vi "Query Current.vi"(8 "error in (no error)":errorcluster, 11 "VISA resource name":refnum<visa-resource-name>) -> (0 "error out":errorcluster, 1 "Ch2 Motor current (I)":sgl, 2 "Ch1  Motor current (I)":sgl, 3 "VISA resource name out":refnum<visa-resource-name>, 4 "Ch2 Battery current (I)":sgl, 5 "Motor Currents":T1, 6 "Ch1 Battery current (I)":sgl)   [LabVIEW 2011, in "Roboteq.lvlib"]
uses:
  Roboteq.lvlib
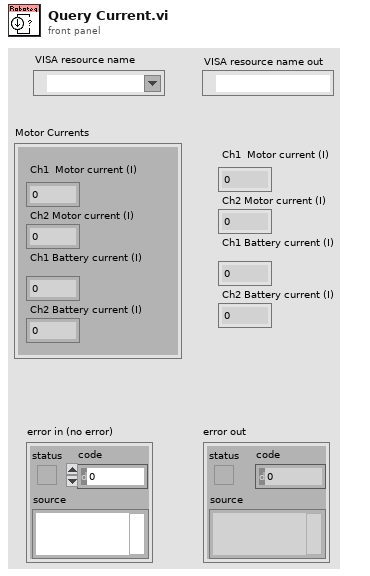
[diagram p1: front panel]
types:
  T1 = cluster{" Ch1  Motor current (I)":sgl, " Ch2 Motor current (I)":sgl, " Ch1 Battery current (I)":sgl, " Ch2 Battery current (I)":sgl}
  T2 = cluster{" Ch1  Motor current (I)":sgl, " Ch2 Motor current (I)":sgl, " Ch1 Battery current (I)":sgl, " Ch2 Battery current (I) 2":sgl}
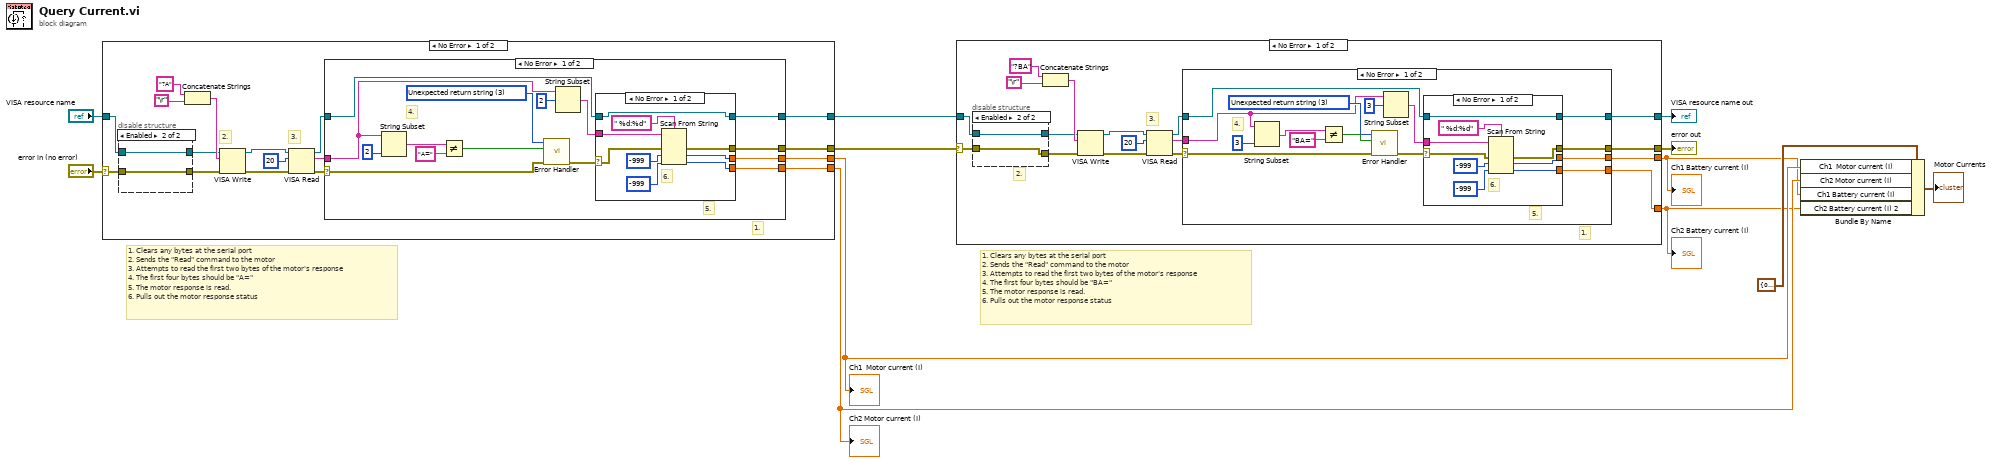
[diagram p0: block diagram]
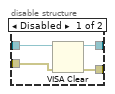
[diagram p2: hidden frame]
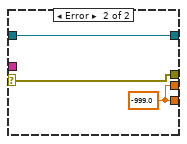
[diagram p3: hidden frame]
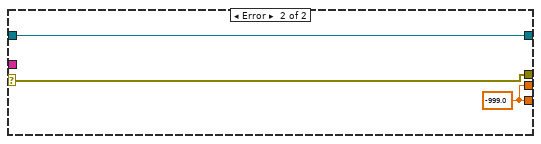
[diagram p4: hidden frame]
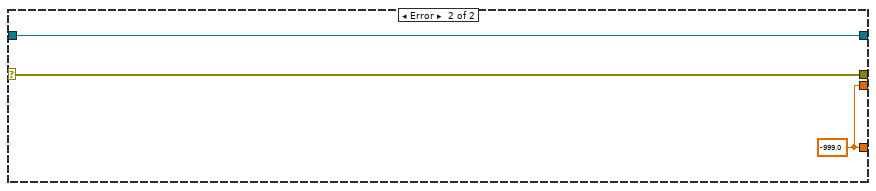
[diagram p5: hidden frame]
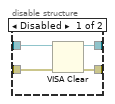
[diagram p6: hidden frame]
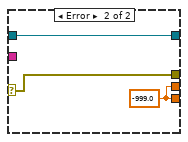
[diagram p7: hidden frame]
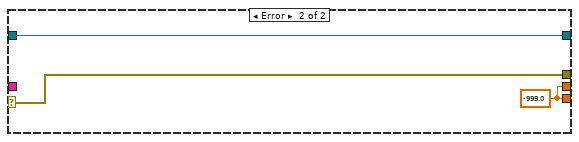
[diagram p8: hidden frame]
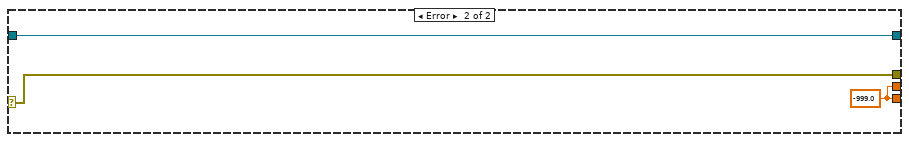
[diagram p9: hidden frame]
diagram:
  # "1. Clears any bytes at the serial port\n2. Sends the \"Read\" command to the motor\n3. Attempts to read the first two bytes of the motor's response\n4. The first four bytes should be \"BA=\"\n5. The motor response is read.\n6. Pulls out the motor response status"
  # "1. Clears any bytes at the serial port\n2. Sends the \"Read\" command to the motor\n3. Attempts to read the first two bytes of the motor's response\n4. The first four bytes should be \"A=\"\n5. The motor response is read.\n6. Pulls out the motor response status"
  n1 = case shown="No Error" "error in (no error)" {
    selector: "error in (no error)" -> [w15 w68]
    tunnel: [w18 w68] -> w9
    tunnel: [w19 w67] -> w3
    tunnel: [w20 w67] -> w4
    tunnel: "VISA resource name" -> [w16 w66]
    tunnel: [w17 w66] -> w10
    frame No Error {
      # "1."
      # "3."
      # "2."
      n2 = disable-structure shown="Enabled" {
        disable-tunnel: w16 -> [w30 w35]
        disable-tunnel: w15 -> [w33 w34]
        disable-tunnel: [w32 w35] -> w14
        disable-tunnel: [w31 w34] -> w13
        frame Disabled {
          n3 = VISA Clear(VISA resource name=w30, error in (no error)=w33) -> (VISA resource name out=w32:refnum<visa-resource-name>, error out=w31:errorcluster)
        }
        frame Enabled {
        }
      }
      n4 = Concatenate Strings("?A" ("string"), "\r") -> (w28:string)
      n5 = VISA Write(VISA resource name=w14, write buffer=w28, error in (no error)=w13) -> (VISA resource name out=w25:refnum<visa-resource-name>, error out=w24:errorcluster)  [unwired: 1 out]
      n6 = VISA Read(VISA resource name=w25, byte count=u32 20, error in (no error)=w24) -> (VISA resource name out=w22:refnum<visa-resource-name>, read buffer=w21:string, error out=w23:errorcluster)  [unwired: 1 out]
      n7 = case shown="No Error" w23 {
        selector: w23 -> [w46 w65]
        tunnel: w21 -> [w38 _]
        tunnel: [w48 w65] -> w18
        tunnel: w22 -> [w50 w64]
        tunnel: [w49 w64] -> w17
        tunnel: [w42 w63] -> w20
        tunnel: [w41 w63] -> w19
        frame No Error {
          w43 = u16 3 items=["Scan timeout"=1, "Invalid motor checksum"=2, "Unexpected return string"=3, "Invalid address range"=4] ("Error type")
          # "5."
          # "4."
          n8 = String Subset(string=w38, length (rest)=2 ("length (rest)")) -> (substring=w39:string)  [unwired: 1 in]
          n9 = Not Equal?(x=w39, y="A=" ("string")) -> (x != y?=w45:bool)
          n10 = call "Error Handler.vi"("error in (no error)"=w46, "Error? (no error)"=w45, "Error type"=w43) -> ("error out"=w47:errorcluster)  [unwired: 8 in]
          n11 = String Subset(string=w38, offset (0)=2 ("length (rest)")) -> (substring=w36:string)  [unwired: 1 in]
          n12 = case shown="No Error" w47 {
            selector: w47 -> [w54 w62]
            tunnel: w36 -> [w55 _]
            tunnel: [w53 w62] -> w48
            tunnel: [w59 w61] -> w49
            tunnel: w50 -> [w59 w61]
            tunnel: [w52 w60] -> w42
            tunnel: [w51 w60] -> w41
            frame No Error {
              # "6."
              n13 = Scan From String(format string=" %d:%d", input string=w55, error in=w54, default 1=-999 ("default value 1"), default 2=-999 ("default value 1")) -> (error out=w53:errorcluster, output 1=w52:i32, output 2=w51:i32)  [unwired: 1 in, 2 out]
            }
            frame Error {
              w60 = sgl -999.0 ("main battery\nvoltage (V)")
            }
          }
        }
        frame Error {
          w63 = sgl -999.0 ("main battery\nvoltage (V)")
        }
      }
    }
    frame Error {
      w67 = sgl -999.0 ("main battery\nvoltage (V)")
    }
  }
  "Ch1  Motor current (I)" <- w4
  "Ch2 Motor current (I)" <- w3
  n14 = case shown="No Error" w9 {
    selector: w9 -> [w71 w124]
    tunnel: [w74 w124] -> w7
    tunnel: [w75 w123] -> w1
    tunnel: [w76 w123] -> w2
    tunnel: w10 -> [w72 w122]
    tunnel: [w73 w122] -> w8
    frame No Error {
      # "1."
      # "3."
      # "2."
      n15 = disable-structure shown="Enabled" {
        disable-tunnel: w72 -> [w89 w91]
        disable-tunnel: w71 -> [w88 w90]
        disable-tunnel: [w87 w91] -> w70
        disable-tunnel: [w86 w90] -> w69
        frame Disabled {
          n16 = VISA Clear(VISA resource name=w89, error in (no error)=w88) -> (VISA resource name out=w87:refnum<visa-resource-name>, error out=w86:errorcluster)
        }
        frame Enabled {
        }
      }
      n17 = Concatenate Strings("?BA" ("string"), "\r") -> (w84:string)
      n18 = VISA Write(VISA resource name=w70, write buffer=w84, error in (no error)=w69) -> (VISA resource name out=w81:refnum<visa-resource-name>, error out=w80:errorcluster)  [unwired: 1 out]
      n19 = VISA Read(VISA resource name=w81, byte count=u32 20, error in (no error)=w80) -> (VISA resource name out=w78:refnum<visa-resource-name>, read buffer=w77:string, error out=w79:errorcluster)  [unwired: 1 out]
      n20 = case shown="No Error" w79 {
        selector: w79 -> [w102 w121]
        tunnel: w77 -> [w94 _]
        tunnel: [w104 w121] -> w74
        tunnel: w78 -> [w106 w120]
        tunnel: [w105 w120] -> w73
        tunnel: [w98 w119] -> w76
        tunnel: [w97 w119] -> w75
        frame No Error {
          w99 = u16 3 items=["Scan timeout"=1, "Invalid motor checksum"=2, "Unexpected return string"=3, "Invalid address range"=4] ("Error type")
          # "5."
          # "4."
          n21 = String Subset(string=w94, length (rest)=3 ("length (rest)")) -> (substring=w95:string)  [unwired: 1 in]
          n22 = Not Equal?(x=w95, y="BA=" ("string")) -> (x != y?=w101:bool)
          n23 = call "Error Handler.vi"("error in (no error)"=w102, "Error? (no error)"=w101, "Error type"=w99) -> ("error out"=w103:errorcluster)  [unwired: 8 in]
          n24 = String Subset(string=w94, offset (0)=3 ("length (rest)")) -> (substring=w92:string)  [unwired: 1 in]
          n25 = case shown="No Error" w103 {
            selector: w103 -> [w110 w118]
            tunnel: w92 -> [w111 _]
            tunnel: [w109 w118] -> w104
            tunnel: [w115 w117] -> w105
            tunnel: w106 -> [w115 w117]
            tunnel: [w108 w116] -> w98
            tunnel: [w107 w116] -> w97
            frame No Error {
              # "6."
              n26 = Scan From String(format string=" %d:%d", input string=w111, error in=w110, default 1=-999 ("default value 1"), default 2=-999 ("default value 1")) -> (error out=w109:errorcluster, output 1=w108:i32, output 2=w107:i32)  [unwired: 1 in, 2 out]
            }
            frame Error {
              w116 = sgl -999.0 ("main battery\nvoltage (V)")
            }
          }
        }
        frame Error {
          w119 = sgl -999.0 ("main battery\nvoltage (V)")
        }
      }
    }
    frame Error {
      w123 = sgl -999.0 ("main battery\nvoltage (V)")
    }
  }
  "VISA resource name out" <- w8
  "error out" <- w7
  "Ch2 Battery current (I)" <- w1
  "Ch1 Battery current (I)" <- w2
  n27 = Bundle By Name(cluster=T2 {" Ch1  Motor current (I)"=0.0, " Ch2 Motor current (I)"=0.0, " Ch1 Battery current (I)"=0.0, " Ch2 Battery current (I) 2"=0.0} ("Motor Currents"), "Ch1  Motor current (I)"=w4, "Ch2 Motor current (I)"=w3, "Ch1 Battery current (I)"=w2, "Ch2 Battery current (I) 2"=w1) -> (→"Motor Currents":T2)
